vi "ST5520_CMD.vi"() -> (2 "DATA FINALE":string)   [LabVIEW 2020]
uses:
  <vilib>/Instr/_visa.llb/VISA Find Search Mode.ctl
panel:
  out "errout":errorcluster caption="sortie d'erreur"
  in  "Arrêter":bool
  in  "errin":errorcluster caption="entrée d'erreur (pas d'erreur)"
  out "VISA OUT":refnum<visa-resource-name>
  out "DATA LIVE":string
  # "DATA OUT"
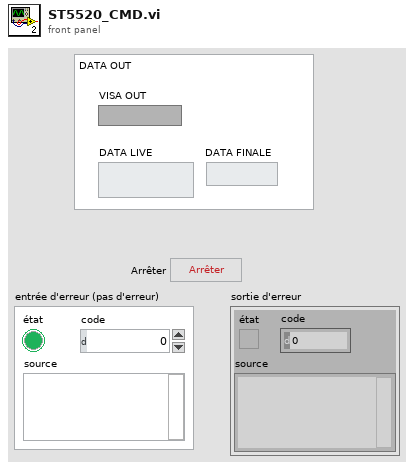
[diagram p1: front panel]
types:
  T1 = typedef "VISA Find Search Mode.ctl" = u32
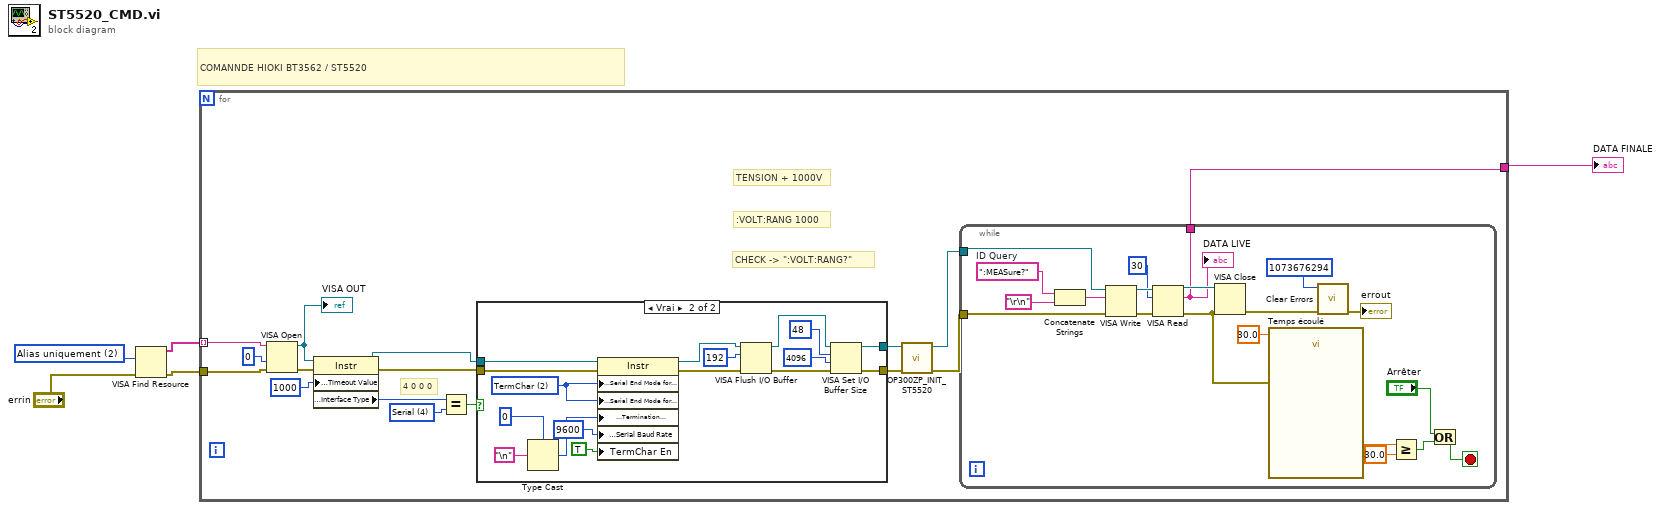
[diagram p0: block diagram]
diagram:
  w5 = T1 2 items=["Noms canoniques uniquement"=0, "Alias uniquement"=2, "Inclure les alias correspondants"=3, "Inclure tous les alias"=4] ("Search Mode")
  # "COMANNDE HIOKI BT3562 / ST5520"
  n1 = VISA Find Resource(8:"errin", 10:w5) -> (0:w3:errorcluster, 3:w4:string[])  [unwired: 1 in, 1 out]
  n2 = for {
    tunnel: w4 -> [w15] mode=indexing
    tunnel: w3 -> [w14]
    tunnel: [w10] -> w1
    w17 = u16 4 items=["GPIB"=1, "VXI"=2, "GPIB-VXI"=3, "Serial"=4, "PXI"=5, "TCPIP"=6, "USB"=7] ("Interface Information:Interface Type")
    # "CHECK -> \":VOLT:RANG?\""
    # ":VOLT:RANG 1000"
    # "TENSION + 1000V"
    # "4 0 0 0"
    n3 = VISA Open(access mode=u32 0, error in (no error)=w14, VISA resource name=w15) -> (VISA resource name=w19:refnum<visa-resource-name>, error out=w18:errorcluster)  [unwired: 2 in]
    "VISA OUT" <- w19
    n4 = property class="Instr"(reference=w19, error in=w18, "General Settings:Timeout Value"=u32 1000) -> (reference out=w12:refnum<visa-resource-name>, error out=w11:errorcluster, "Interface Information:Interface Type"=w16:u16)
    n5 = Equal?(x=w16, y=w17) -> (x = y?=w13:bool)
    n6 = case shown="Vrai" w13 {
      tunnel: [w42 w57] -> w8
      tunnel: [w43 w54] -> w9
      tunnel: w12 -> [w42 w59]
      tunnel: w11 -> [w43 w60]
      frame False {
        # "EDIT: Remove interfaces not supported by your instrument."
        # "GPIB, TCP/IP, and USB Interface"
      }
      frame True {
        w47 = u16 2 items=["None", "LastBit", "TermChar"] ("Serial Settings:Serial End Mode for Reads")
        n7 = Type Cast(type=u8 0, x="\n" ("Line Feed Constant")) -> (*(type *) &x=w46:u8)
        n8 = property class="Instr"(reference=w59, error in=w60, "Serial Settings:Serial End Mode for Reads"=w47, "Serial Settings:Serial End Mode for Writes"=w47, "Message Based Settings:Termination Character"=w46, "Serial Settings:Serial Baud Rate"=u32 9600 ("Serial Settings:Baud Rate"), "TermChar En"=TRUE ("Message Based Settings:Termination Character Enable")) -> (reference out=w53:refnum<visa-resource-name>, error out=w56:errorcluster)
        n9 = VISA Flush I/O Buffer(VISA resource name=w53, mask (16)=u16 192, error in (no error)=w56) -> (VISA resource name out=w58:refnum<visa-resource-name>, error out=w55:errorcluster)
        n10 = VISA Set I/O Buffer Size(VISA resource name=w58, mask (16)=u16 48, size (4096)=u32 4096 ("size (0)"), error in (no error)=w55) -> (VISA resource name out=w57:refnum<visa-resource-name>, error out=w54:errorcluster)
      }
    }
    n11 = call "OP300ZP_INIT_ST5520.vi"("entrée d'erreur (pas d'erreur)"=w9, "VISA"=w8) -> ("sortie d'erreur"=w6:errorcluster, "VISA"=w7:refnum<visa-resource-name>)  [unwired: 8 in]
    n12 = while {
      tunnel: w6 -> [w32]
      tunnel: w7 -> [w33]
      tunnel: [w22] -> w10
      stop <- w23 stop-if-true
      w41 = ":MEASure?"  # ID Query
      n13 = Concatenate Strings(w41, "\r\n") -> (w35:string)
      n14 = VISA Write(VISA resource name=w33, write buffer=w35, error in (no error)=w32) -> (VISA resource name out=w40:refnum<visa-resource-name>, error out=w39:errorcluster)  [unwired: 1 out]
      n15 = VISA Read(VISA resource name=w40, byte count=u32 30 ("nombre d'octets"), error in (no error)=w39) -> (VISA resource name out=w37:refnum<visa-resource-name>, read buffer=w22:string, error out=w28:errorcluster)  [unwired: 1 out]
      "DATA LIVE" <- w22
      n16 = VISA Close(VISA resource name=w37, error in (no error)=w28) -> (error out=w38:errorcluster)
      n17 = call "Temps écoulé"("Time Target (s)"=30.0, "error in (no error)"=w28) -> ("Elapsed Time (s)"=w27:dbl)  [unwired: 10 in, 7 out]
      n18 = call <vilib>:"Clear Errors.vi"("error in (no error)"=w38, "specific error code to clear (0: all)"=1073676294) -> ("error out"=→"errout":errorcluster)  [unwired: 4 in, 1 out]
      n19 = Greater Or Equal?(x=w27, y=30.0) -> (x >= y?=w25:bool)
      n20 = Or(x="Arrêter", y=w25) -> (x .or. y?=w23:bool)
    }
  }
  "DATA FINALE" <- w1
